vi "Read Data.vi"(7 "Data Block":u16, 8 "error in (no error)":errorcluster, 9 "Default Data":variant, 10 "Start Address":u32, 11 "SIMATIC_S7 in":refnum<class "SIMATIC_S7.lvclass">) -> (0 "error out":errorcluster, 2 "Data":variant, 3 "SIMATIC_S7 out":refnum<class "SIMATIC_S7.lvclass">)   [LabVIEW 2025, in "SIMATIC_S7.lvclass"]
uses:
  SIMATIC_S7.lvclass
  SIMATIC_S7.lvclass/SIMATIC_S7.ctl
  <vilib>/Utility/Data Type/NI_Data Type.lvlib
  <vilib>/Hampel Software Engineering/S7NetCom/Source/S7NetCom.lvclass
  <vilib>/Hampel Software Engineering/S7NetCom/Source/Controls/S7_Memory_Area.ctl
  <vilib>/Hampel Software Engineering/S7NetCom/Source/API/Read Data - Byte (Scalar).vi
  <vilib>/Hampel Software Engineering/S7NetCom/Source/API/Read Data - Byte (Array).vi
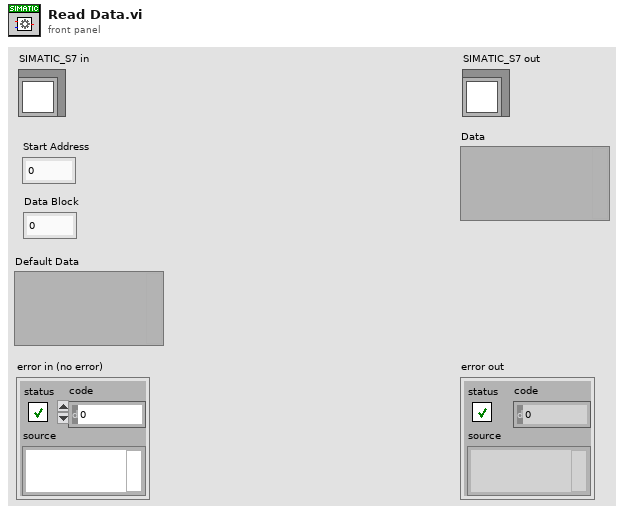
[diagram p1: front panel]
types:
  T1 = typedef "S7NetCom.lvlib/S7NetCom.lvclass/S7_Memory_Area.ctl" = enum8{"P Area", "I Area", "O Area", "M Area", "DB Area", "Counter", "Timer"}
  T2 = typedef "NI_Data Type.lvlib/Data Type.ctl" = enum8{"Invalid Type", "Void", "I8", "I16", "I32", "I64", "U8", "U16", "U32", "U64", "Single Float", "Double Float", "Extended Float", "Single Complex", "Double Complex", "Extended Complex", "Enum U8", "Enum U16", "Enum U32", "Enum U64", "Single Float With Unit", "Double Float With Unit", "Extended Float With Unit", "Single Complex with Unit", "Double Complex with Unit", "Extended Complex with Unit", "Boolean", "String", "Path", "Picture", "Tag", "Array", "Cluster", "Variant", "LV Variant", "Waveform", "Timestamp", "Digital Waveform", "Digital Data", "ExpressData", "Refnum", "External Data", "VI", "Poly VI", "LabVIEW Class Instance", "Fixed Point", "Set Collection", "Map Collection"}
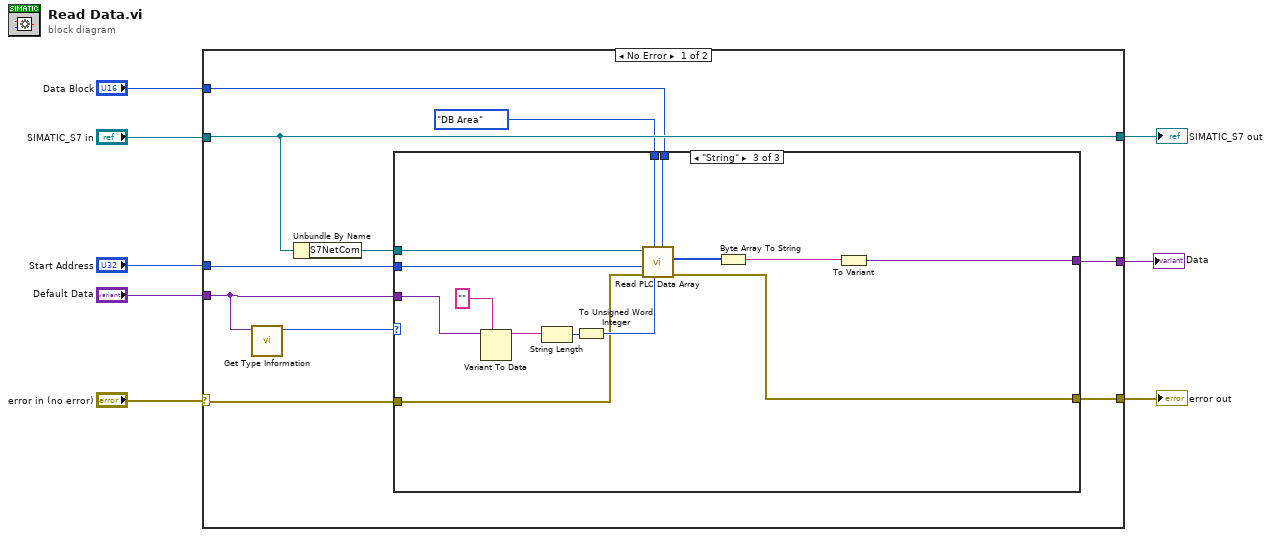
[diagram p0: block diagram]
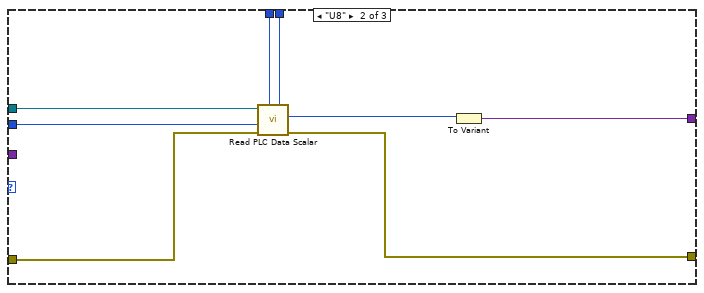
[diagram p3: hidden frame]
diagram:
  n1 = case shown="No Error" "error in (no error)" {
    selector: "error in (no error)" -> [w14 w43]
    tunnel: "SIMATIC_S7 in" -> [w18 w45]
    tunnel: [w18 w45] -> w6
    tunnel: "Data Block" -> [w10 _]
    tunnel: "Start Address" -> [w9 _]
    tunnel: "Default Data" -> [w11 w44]
    tunnel: [w15 w44] -> w2
    tunnel: [w13 w43] -> w1
    frame No Error {
      n2 = call <vilib>:"Get Type Information.vi"("variant"=w11) -> ("type"=w17:T2)  [unwired: 6 in, 4 out]
      n3 = Unbundle By Name(w18) -> ("S7NetCom"=w16:refnum<class "S7NetCom.lvclass">)
      n4 = case shown="\"String\"" w17 {
        tunnel: w16 -> [_ w28 w38]
        tunnel: [w20 w26 w42] -> w15
        tunnel: w14 -> [w19 w25 w30]
        tunnel: [w19 w24 w29] -> w13
        tunnel: S7_Memory_Area."DB Area" ("Memory Area") -> [_ w23 w37]
        tunnel: w11 -> [w20 _ w41]
        tunnel: w10 -> [_ w22 w36]
        tunnel: w9 -> [_ w21 w35]
        frame Default {
        }
        frame "U8" {
          n5 = call-poly <vilib>:"Read PLC Data Scalar.vi"("Data Block #"=w22, "Memory Area"=w23, "error in (no error)"=w25, "Start Address"=w21, "S7 in"=w28) -> ("error out"=w24:errorcluster, "Byte Value"=w27:u8)  [unwired: 4 in, 1 out]
          n6 = To Variant(anything=w27) -> (Variant=w26:variant)
        }
        frame "String" {
          n7 = Variant To Data(type="", Variant=w41) -> (data=w39:string)  [unwired: 1 in, 1 out]
          n8 = String Length(string=w39) -> (length=w34:i32)
          n9 = To Unsigned Word Integer(number=w34) -> (unsigned 16bit integer=w33:u16)
          n10 = call-poly <vilib>:"Read PLC Data Array.vi"("Data Block #"=w36, "Read Length"=w33, "Memory Area"=w37, "error in (no error)"=w30, "Start Address"=w35, "S7 in"=w38) -> ("error out"=w29:errorcluster, "Byte Array"=w32:u8[])  [unwired: 3 in, 1 out]
          n11 = Byte Array To String(unsigned byte array=w32) -> (string=w31:string)
          n12 = To Variant(anything=w31) -> (Variant=w42:variant)
        }
      }
    }
    frame Error {
    }
  }
  "error out" <- w1
  "SIMATIC_S7 out" <- w6
  "Data" <- w2
